vi "Write Shift Status.vi"(10 "Gear":T1, 11 "Autoshifting":bool) -> (3 "Shift Status":dbl)   [LabVIEW 2017]
uses:
  <vilib>/Rock Robotics/WPI/Solenoid/WPI_SolenoidValue.ctl
  <vilib>/Rock Robotics/Network Tables/NT Write Number.vi
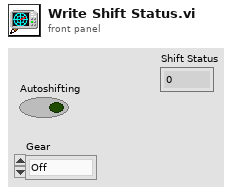
[diagram p1: front panel]
types:
  T1 = typedef "WPI_SolenoidValue.ctl" = enum16{"Off", "On", "Forward", "Reverse"}
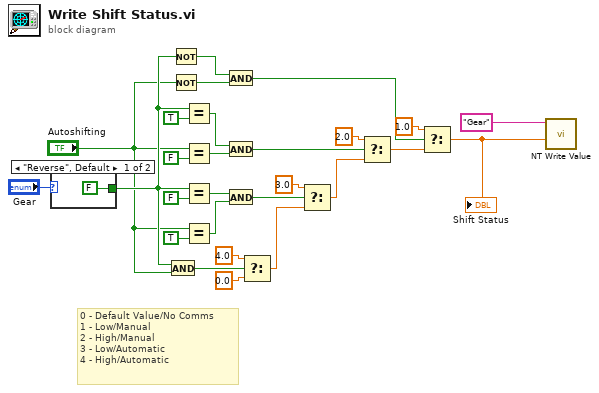
[diagram p0: block diagram]
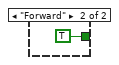
[diagram p2: hidden frame]
diagram:
  # "0 - Default Value/No Comms\n1 - Low/Manual\n2 - High/Manual\n3 - Low/Automatic\n4 - High/Automatic"
  n1 = case shown="\"Reverse\", Default" "Gear" {
    tunnel: [FALSE TRUE] -> w3
    frame "Reverse", Default {
    }
    frame "Forward" {
    }
  }
  n2 = And(x=w3, y="Autoshifting") -> (x .and. y?=w1:bool)
  n3 = Not(x=w3) -> (.not. x?=w5:bool)
  n4 = Not(x="Autoshifting") -> (.not. x?=w6:bool)
  n5 = Equal?(x=w3, y=TRUE) -> (x = y?=w24:bool)
  n6 = Equal?(x="Autoshifting", y=FALSE) -> (x = y?=w22:bool)
  n7 = Equal?(x=w3, y=FALSE) -> (x = y?=w14:bool)
  n8 = Equal?(x="Autoshifting", y=TRUE) -> (x = y?=w13:bool)
  n9 = And(x=w5, y=w6) -> (x .and. y?=w4:bool)
  n10 = And(x=w24, y=w22) -> (x .and. y?=w23:bool)
  n11 = And(x=w14, y=w13) -> (x .and. y?=w15:bool)
  n12 = Select(t=4.0, s=w1, f=0.0) -> (s? t:f=w10:dbl)
  n13 = Select(t=3.0, s=w15, f=w10) -> (s? t:f=w12:dbl)
  n14 = Select(t=2.0, s=w23, f=w12) -> (s? t:f=w19:dbl)
  n15 = Select(t=1.0, s=w4, f=w19) -> (s? t:f=w8:dbl)
  "Shift Status" <- w8
  n16 = call-poly <vilib>:"NT Write Value.vi"("Numeric"=w8, "Name"="Gear") -> ()  [unwired: 9 in, 1 out]
